vi "Configure Serial Bus (SENT - Basic).vi"(0 "VISA resource name":refnum<visa-resource-name>, 5 "Serial Bus Name (1: Serial Bus 1)":u16(ring)=1 items=["Serial Bus 1"=1, "Serial Bus 2"=2], 7 "Input Source (1: Channel 1)":i32(ring)=1 items=["Channel 1"=1, "Channel 2"=2, "Channel 3"=3, "Channel 4"=4, "D0"=5, "D1"=6, "D2"=7, "D3"=8, "D4"=9, "D5"=10, "D6"=11, "D7"=12, "D8"=13, "D9"=14, "D10"=15, "D11"=16, "D12"=17, "D13"=18, "D14"=19, "D15"=20], 9 "Message Format (0: Fast Nibbles (All))":u16(ring) items=["Fast Nibbles (All)", "Fast Signals", "Fast + Short Serial", "Fast + Enhanced Serial", "Short Serial", "Enhanced Serial"], 11 "error in (no error)":errorcluster, 12 "Display Format (0: Hex)":u16(ring) items=["Hex", "Decimal", "Symbolic"]) -> (4 "VISA resource name out":refnum<visa-resource-name>, 15 "error out":errorcluster)   [LabVIEW 2015, in "Agilent 2000 3000 X-Series.lvlib"]
doc: "Configures basic parameters for SENT serial decoding.\n\nNote:\nThis VI is not supported by EDUX1052A/G, DSOX1202A/G, DSOX1204A/G models"
uses:
  Agilent 2000 3000 X-Series.lvlib
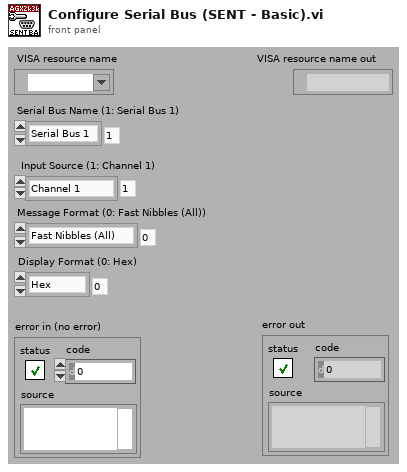
[diagram p1: front panel]
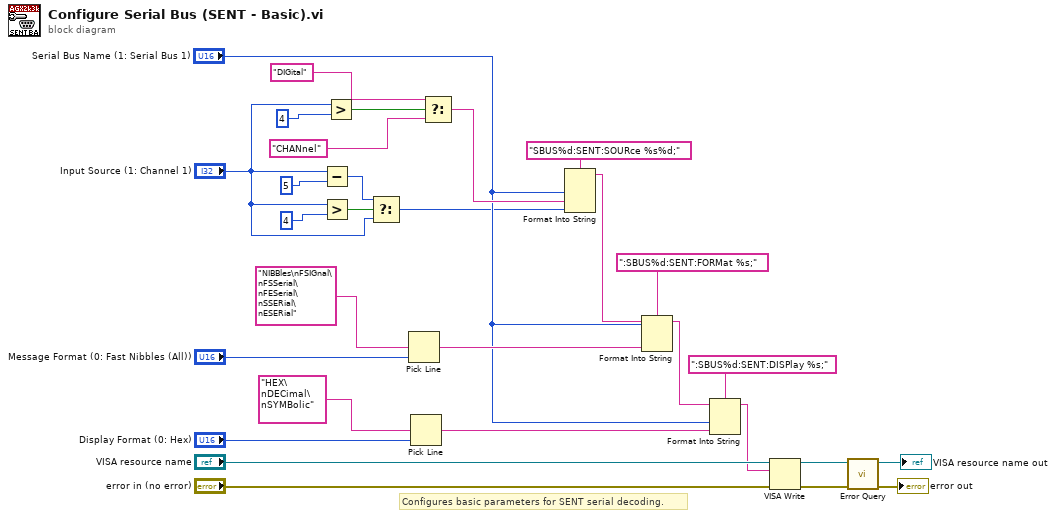
[diagram p0: block diagram]
diagram:
  # "Configures basic parameters for SENT serial decoding."
  n1 = Subtract(x="Input Source (1: Channel 1)", y=5) -> (x-y=w4:i32)
  n2 = Greater?(x="Input Source (1: Channel 1)", y=4) -> (0:w7:bool)
  n3 = Greater?(x="Input Source (1: Channel 1)", y=4) -> (0:w27:bool)
  n4 = Select(t=w4, s=w7, f="Input Source (1: Channel 1)") -> (s? t:f=w3:i32)
  n5 = Pick Line(multi-line string="NIBBles\nFSIGnal\nFSSerial\nFESerial\nSSERial\nESERial", line index="Message Format (0: Fast Nibbles (All))") -> (output string=w22:string)  [unwired: 1 in]
  n6 = Pick Line(multi-line string="HEX\nDECimal\nSYMBolic", line index="Display Format (0: Hex)") -> (output string=w15:string)  [unwired: 1 in]
  n7 = Select(t="DIGital" ("f"), s=w27, f="CHANnel") -> (s? t:f=w25:string)
  n8 = Format Into String(format string="SBUS%d:SENT:SOURce %s%d;", "Serial Bus Name (1: Serial Bus 1)", w25, w3) -> (resulting string=w20:string)  [unwired: 2 in, 1 out]
  n9 = Format Into String(format string=":SBUS%d:SENT:FORMat %s;", initial string=w20, "Serial Bus Name (1: Serial Bus 1)", w22) -> (resulting string=w19:string)  [unwired: 1 in, 1 out]
  n10 = Format Into String(format string=":SBUS%d:SENT:DISPlay %s;", initial string=w19, "Serial Bus Name (1: Serial Bus 1)", w15) -> (resulting string=w14:string)  [unwired: 1 in, 1 out]
  n11 = VISA Write(VISA resource name="VISA resource name", write buffer=w14, error in (no error)="error in (no error)") -> (VISA resource name out=w13:refnum<visa-resource-name>, error out=w12:errorcluster)  [unwired: 1 out]
  n12 = call "Error Query.vi"("error in (no error)"=w12, "VISA resource name"=w13) -> ("error out"=→"error out":errorcluster, "VISA resource name out"=→"VISA resource name out":refnum<visa-resource-name>)  [unwired: 6 in, 2 out]
